vi "Status SpecimenTempCtrlParameter.vi"(8 "error in (no error)":errorcluster, 10 "Address (0)":i32, 11 "VISA resource name":refnum<visa-resource-name>) -> (0 "error out":errorcluster, 2 "Specimen TempCtrl Parameter":T1, 3 "VISA resource name out":refnum<visa-resource-name>)   [LabVIEW 2016, in "Environment Chamber.lvlib" / "Climatic Chamber.lvlib"]
doc: "<b>Specimen temperature control parameter monitor</B>\n\nReturns the setting parameter related to specimen temperature control."
uses:
  Climatic Chamber.lvlib
  Private/Type Defs/Specimen TempCtrl Settings Cluster.ctl
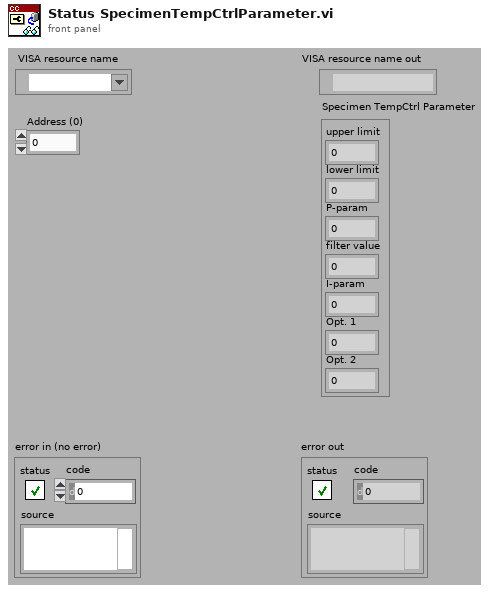
[diagram p1: front panel]
types:
  T1 = typedef "Environment Chamber.lvlib/Climatic Chamber.lvlib/Specimen TempCtrl Settings Cluster.ctl" = cluster{"upper limit":dbl, "lower limit":dbl, "P-param":dbl, "filter value":dbl, "I-param":dbl, "Opt. 1":dbl, "Opt. 2":dbl}
  T2 = cluster{"Array Data[0]":dbl, "Array Data[1]":dbl, "Array Data[2]":dbl, "Array Data[3]":dbl, "Array Data[4]":dbl, "Array Data[5]":dbl, "Array Data[6]":dbl}
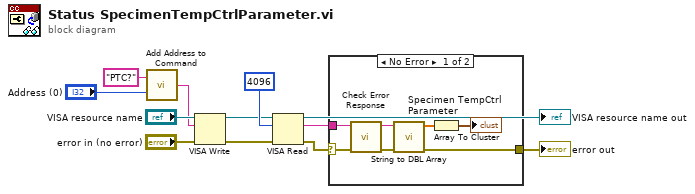
[diagram p0: block diagram]
diagram:
  n1 = call "Add Address to Command.vi"("Address (0)"="Address (0)", "Command"="PTC?") -> ("Command OUT"=w5:string)
  n2 = VISA Write(VISA resource name="VISA resource name", write buffer=w5, error in (no error)="error in (no error)") -> (VISA resource name out=w9:refnum<visa-resource-name>, error out=w8:errorcluster)  [unwired: 1 out]
  n3 = VISA Read(VISA resource name=w9, byte count=u32 4096, error in (no error)=w8) -> (VISA resource name out=→"VISA resource name out":refnum<visa-resource-name>, read buffer=w3:string, error out=w4:errorcluster)  [unwired: 1 out]
  n4 = case shown="No Error" w4 {
    selector: w4 -> [w18 w20]
    tunnel: w3 -> [w19 _]
    tunnel: [w15 w20] -> w2
    frame No Error {
      n5 = call "Check Error Response.vi"("error in (no error)"=w18, "read String"=w19) -> ("error out"=w17:errorcluster, "String out"=w16:string)  [unwired: 7 in, 1 out]
      n6 = call "String to DBL Array.vi"("error in (no error)"=w17, "String received"=w16) -> ("error out"=w15:errorcluster, "Array Data"=w14:dbl[])  [unwired: 8 in]
      n7 = Array To Cluster(array=w14) -> (cluster=→"Specimen TempCtrl Parameter":T2)
    }
    frame Error {
    }
  }
  "error out" <- w2
